vi "test-SyncMessageWithAttribute.vi"(8 "error in (no error)":errorcluster, 11 "TestCase in":refnum<class "testcase-CSMSyncMessage.lvclass">) -> (0 "error out":errorcluster, 3 "TestCase out":refnum<class "testcase-CSMSyncMessage.lvclass">)   [LabVIEW 2017, in "testcase-CSMSyncMessage.lvclass"]
uses:
  testcase-CSMSyncMessage.lvclass
  src/user.lib/_NEVSTOP/Communicable State Machine(CSM)/AdvanceAPI/CSM - Make String Arguments Safe.vi
  src/user.lib/_NEVSTOP/Communicable State Machine(CSM)/AdvanceAPI/CSM - Keywords.vi
  <vilib>/addons/_JKI Toolkits/VI Tester/TestCase.llb/TestCase.lvclass
  src/user.lib/_NEVSTOP/Communicable State Machine(CSM)/Communicable State Machine.lvlib
  C:/Program Files (x86)/National Instruments/LabVIEW 2017/vi.lib/addons/_JKI Toolkits/VI Tester/TestCase.llb/TestCase.lvclass
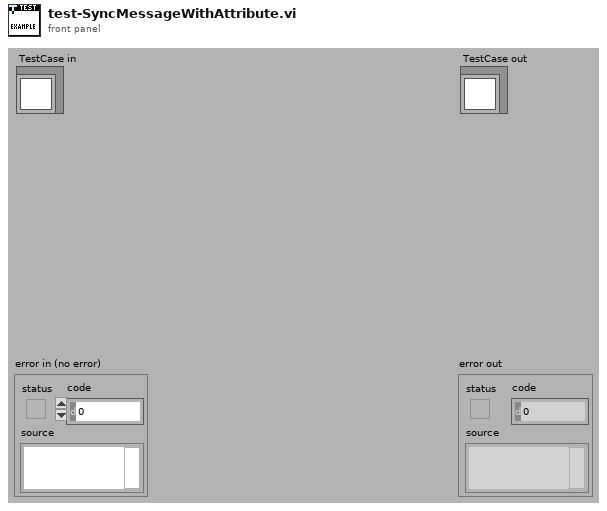
[diagram p1: front panel]
types:
  T1 = cluster{"Arguments":string, "Response":string, "error":errorcluster}
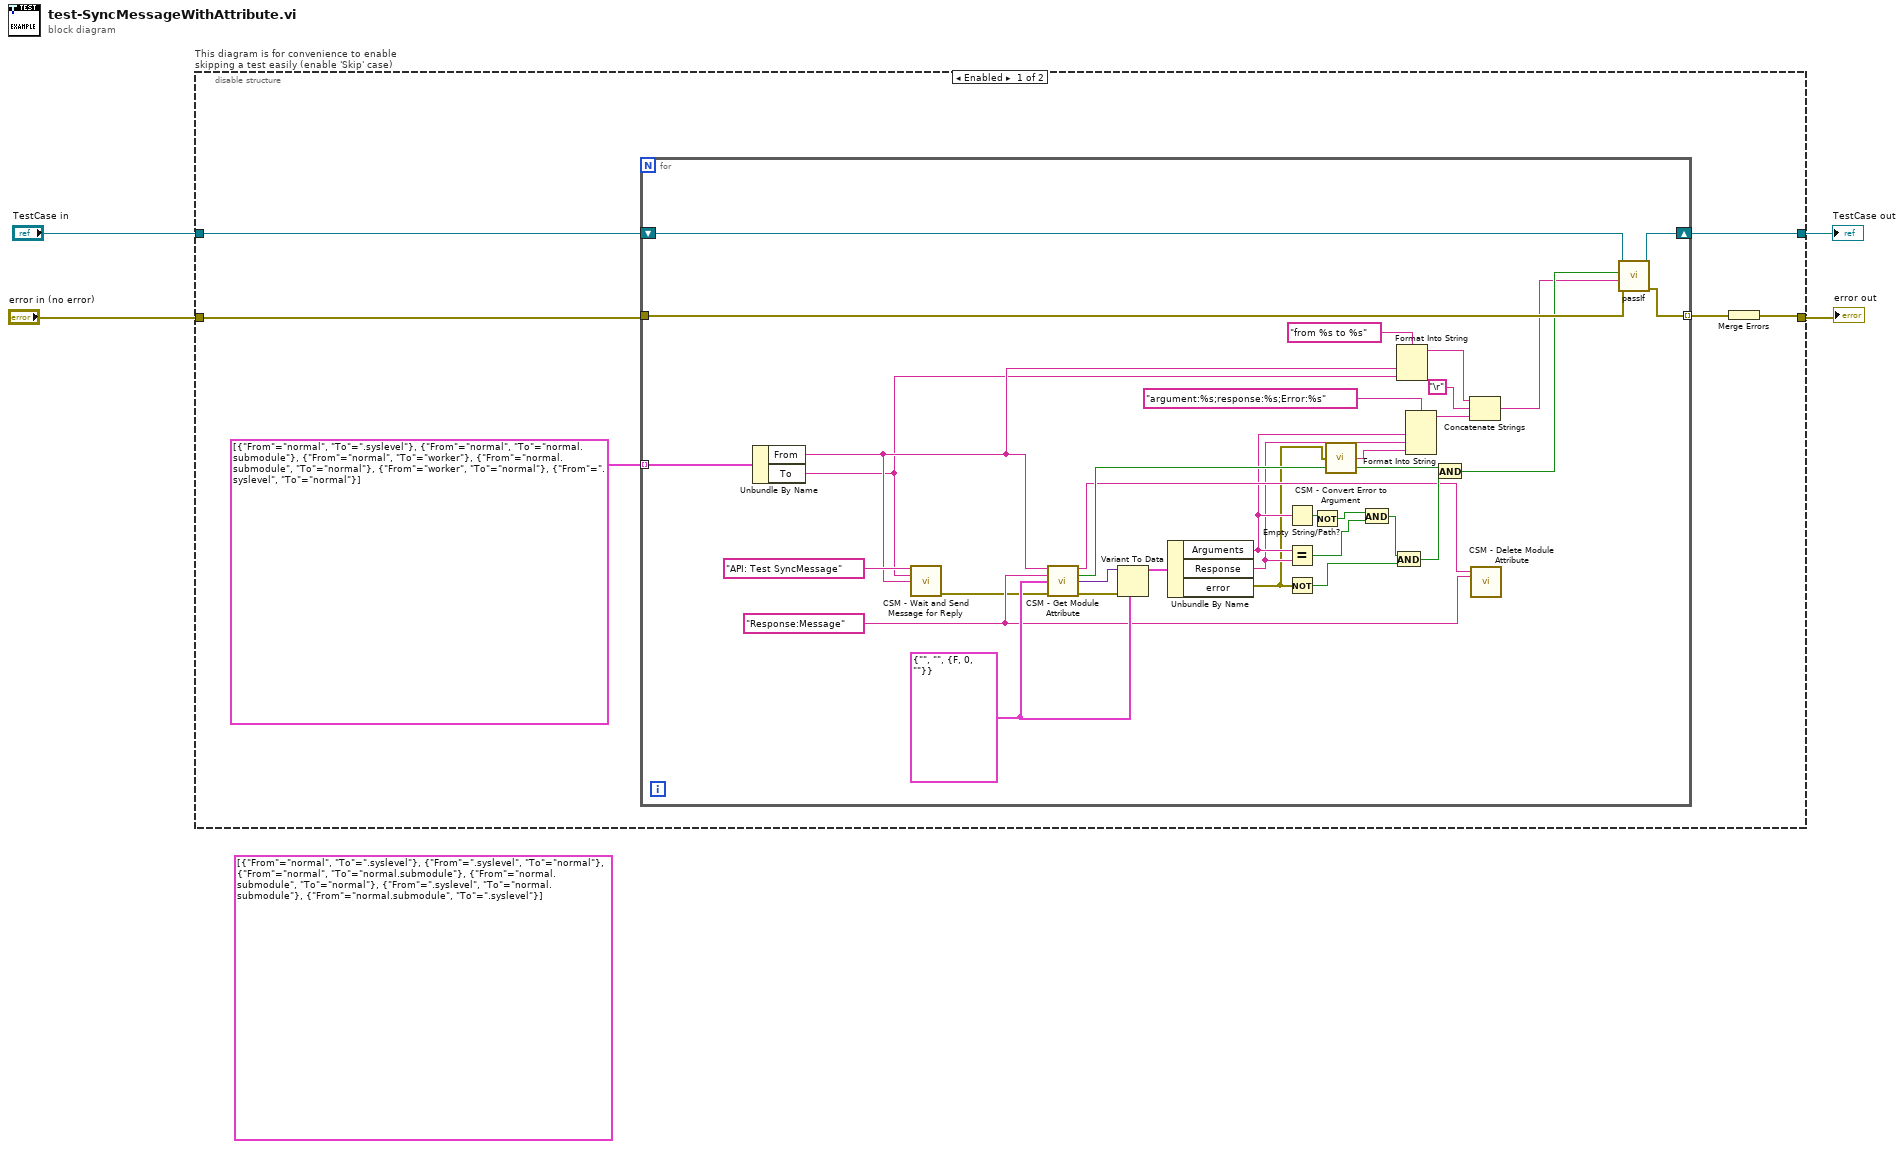
[diagram p0: block diagram]
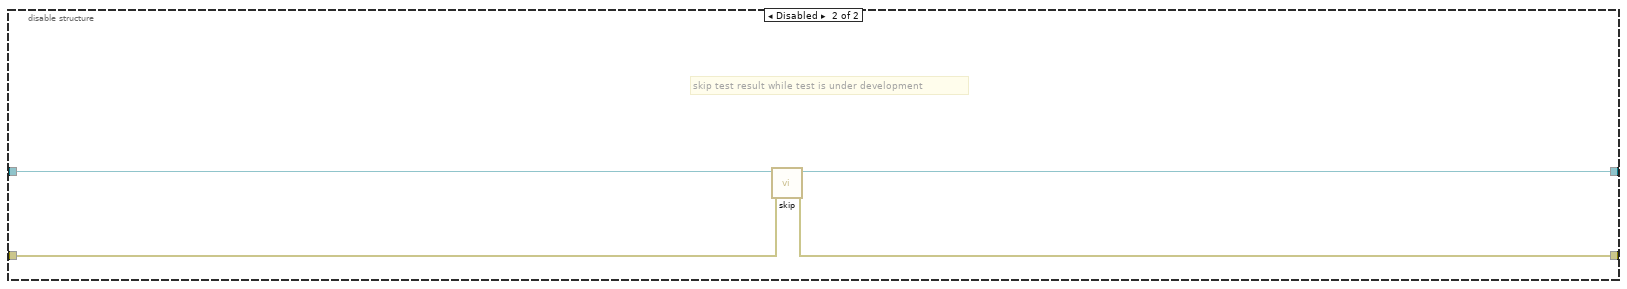
[diagram p2: hidden frame]
diagram:
  (unwired) cluster{"From":string, "To":string}[] [{"From"="normal", "To"=".syslevel"}, {"From"=".syslevel", "To"="normal"}, {"From"="normal", "To"="normal.submodule"}, {"From"="normal.submodule", "To"="normal"}, {"From"=".syslevel", "To"="normal.submodule"}, {"From"="normal.submodule", "To"=".syslevel"}]
  n1 = disable-structure "This diagram is for convenience to enable skipping a test easily (enable 'Skip' case)" shown="Enabled" {
    disable-tunnel: "TestCase in" -> [w10 w47]
    disable-tunnel: [w9 w45] -> w1
    disable-tunnel: [w5 w46] -> w3
    disable-tunnel: "error in (no error)" -> [w7 w44]
    frame Enabled {
      n2 = for {
        tunnel: cluster{"From":string, "To":string}[] [{"From"="normal", "To"=".syslevel"}, {"From"="normal", "To"="normal.submodule"}, {"From"="normal", "To"="worker"}, {"From"="normal.submodule", "To"="normal"}, {"From"="worker", "To"="normal"}, {"From"=".syslevel", "To"="normal"}] -> [w30] mode=indexing
        shift-right: [w42] -> w9
        shift-left: w10 -> [w43]
        tunnel: w7 -> [w40]
        tunnel: [w41] -> w8 mode=indexing
        w37 = T1 {"Arguments"="", "Response"="", "error"={"status"=FALSE, "code"=0, "source"=""}}
        w25 = "Response:Message" ("State")
        n3 = Unbundle By Name(w30) -> ("From"=w29:string, "To"=w28:string)
        n4 = call "CSM - Wait and Send Message for Reply.vi"("State"="API: Test SyncMessage", "Arguments (\"\")"=w28, "Target Module"=w29) -> ("error out"=w14:errorcluster)  [unwired: 10 in, 2 out]
        n5 = call "CSM - Get Module Attribute.vi"("CSM Name"=w29, "Attribute"=w25, "Default Value (Empty Variant)"=w37, "Error In"=w14) -> ("CSM Name (Dup)"=w26:string, "Found"=w33:bool, "Value"=w36:variant, "error out"=w38:errorcluster)  [unwired: 7 in, 1 out]
        n6 = Variant To Data(error in=w38, type=w37, Variant=w36) -> (data=w35:T1)  [unwired: 1 out]
        n7 = Unbundle By Name(w35) -> ("Arguments"=w20:string, "Response"=w19:string, "error"=w17:errorcluster)
        n8 = Empty String/Path?(string/path=w20) -> (empty?=w24:bool)
        n9 = Equal?(x=w20, y=w19) -> (x = y?=w22:bool)
        n10 = Not(x=w17) -> (.not. x?=w34:bool)
        n11 = Not(x=w24) -> (.not. x?=w23:bool)
        n12 = call "CSM - Convert Error to Argument.vi"("Error"=w17) -> ("Argument"=w18:string)  [unwired: 4 in]
        n13 = And(x=w23, y=w22) -> (x .and. y?=w21:bool)
        n14 = And(x=w21, y=w34) -> (x .and. y?=w32:bool)
        n15 = Format Into String(format string="from %s to %s", w29, w28) -> (resulting string=w12:string)  [unwired: 2 in, 1 out]
        n16 = Format Into String(format string="argument:%s;response:%s;Error:%s", w20, w19, w18) -> (resulting string=w16:string)  [unwired: 2 in, 1 out]
        n17 = And(x=w33, y=w32) -> (x .and. y?=w31:bool)
        n18 = Concatenate Strings(w12, "\r", w16) -> (w13:string)
        n19 = call "CSM - Delete Module Attribute.vi"("CSM Name"=w26, "Attribute"=w25) -> ()  [unwired: 10 in, 4 out]
        n20 = call-dynamic "passIf.vi"("error in (no error)"=w40, "message (\"\")"=w13, "pass"=w31, "TestCase in"=w43) -> ("error out"=w41:errorcluster, "TestCase out"=w42:refnum<class "testcase-CSMSyncMessage.lvclass">)  [unwired: 6 in]
      }
      n21 = Merge Errors(w8) -> (w5:errorcluster)
    }
    frame Disabled {
      # "skip test result while test is under development"
      n22 = call <vilib>:"skip.vi"("error in (no error)"=w44, "TestCase in"=w47) -> ("error out"=w46:errorcluster, "TestCase out"=w45:refnum<class "testcase-CSMSyncMessage.lvclass">)  [unwired: 8 in]
    }
  }
  "error out" <- w3
  "TestCase out" <- w1
